vi "Wait_Main.vi"(4 "Wait time (msec)":u32) -> ()   [LabVIEW 2018]
doc: "Ver 1.00\nREUSEABLE COMPONENT\nDESCRIPTION \nRe-entrant abortable wait. Use within while loops to ensure a quick exit when the stop button is pressed.\n\nERROR HANDLING\nNone\n------------------------------------------------------------------ \nVERSION CONTROL \nVer 1.00 ssdc 20/04/2000"
panel:
  # "Input"
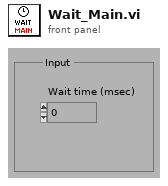
[diagram p1: front panel]
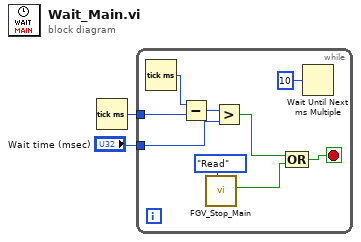
[diagram p0: block diagram]
diagram:
  n1 = Tick Count (ms)() -> (millisecond timer value=w2:u32)
  n2 = while {
    tunnel: "Wait time (msec)" -> [w8]
    tunnel: w2 -> [w11]
    stop <- w6 stop-if-true
    n3 = Tick Count (ms)() -> (millisecond timer value=w10:u32)
    n4 = Subtract(x=w10, y=w11) -> (x-y=w9:u32)
    n5 = call "FGV_Stop_Main.vi"("Action"=enum16{"Read", "Write"}."Read") -> ("Var Out"=w3:bool)  [unwired: 9 in, 1 out]
    n6 = Greater?(x=w9, y=w8) -> (0:w7:bool)
    n7 = Compound Arithmetic op=OR(w7, w3) -> (w6:bool)
    n8 = Wait Until Next ms Multiple(millisecond multiple=u32 10 ("milliseconds to wait")) -> ()  [unwired: 1 out]
  }
